vi "Simulation Time Advance.vi"(8 "error in (no error)":errorcluster, 11 "simulator":T14={"configuration"={"maxTime"=5.0, "enableVisualization"=TRUE, "Environment Definition"=path "irobotNavigationStateMachine.vi", "Record Location"=path "Simulation Record.xml", "autograde?"=TRUE, "interactive?"=FALSE, "Feedback Mode"=enum."debug navigation", "Robot State Charts"=[path "C:/Users/blueuser/Desktop/Robo Sim Berkley/cpsgrader-release-0.4/Simulators/EECS149lab/src/LabVIEW/statechart/Simulation Statechart.vi"], "statechart"=path "C:/Users/blueuser/Desktop/Robo Sim Berkley/cpsgrader-release-0.4/Simulators/EECS149lab/src/LabVIEW/statechart/Simulation Statechart.vi"}, "Statechart\ndisplay"=refnum, "first step?"=FALSE, "Robots Simulation Statecharts"=[], "Robots"=[]}) -> (0 "error out":errorcluster, 2 "Robot Sensors":T1[](array[typedef]) {"Kobuki Sensors"."Infrared" format="%02x"; "iRobot Sensors"."Infrared" format="%02x"; "accelerometer"."z axis (g)" format="%.3f"; "accelerometer"."y axis (g)" format="%.3f"; "accelerometer"."x axis (g)" format="%.3f"}, 3 "simulator":T14={"configuration"={"maxTime"=5.0, "enableVisualization"=TRUE, "Environment Definition"=path "irobotNavigationStateMachine.vi", "Record Location"=path "Simulation Record.xml", "autograde?"=TRUE, "interactive?"=FALSE, "Feedback Mode"=enum."debug navigation", "Robot State Charts"=[path "C:/Users/blueuser/Desktop/Robo Sim Berkley/cpsgrader-release-0.4/Simulators/EECS149lab/src/LabVIEW/statechart/Simulation Statechart.vi"], "statechart"=path "C:/Users/blueuser/Desktop/Robo Sim Berkley/cpsgrader-release-0.4/Simulators/EECS149lab/src/LabVIEW/statechart/Simulation Statechart.vi"}, "Statechart\ndisplay"=refnum, "first step?"=FALSE, "Robots Simulation Statecharts"=[], "Robots"=[]})   [LabVIEW 2014]
uses:
  Simulator.ctl
  CyberSim interface/Simulation Configuration.ctl
  autograder/feedbackMode.ctl
  Multi Bot Code/RobotData.ctl
  <instrlib>/DC Motor Controller/HAIOL/DC Motor Controller.lvclass
  shared/Sensors.ctl
  iRobot/Sensor/Accelerometer.ctl
  iRobot/Sensor/Sensor Group 6.ctl
  iRobot/Sensor/Bumps + Wheel Drops.ctl
  iRobot/Sensor/Buttons.ctl
  iRobot/Sensor/Charging State.ctl
  iRobot/Sensor/Charging Sources Available.ctl
  iRobot/Sensor/OI Mode.ctl
  iRobot/Sensor/Cargo Bay Digital Inputs.ctl
  iRobot/Sensor/Low-Side Driver + Wheel Overcurrent.ctl
  Kobuki/KobukiSensors.ctl
  Kobuki/Kobuki Bumps and WheelDrops.ctl
  Kobuki/Kobuki Buttons.ctl
  <vilib>/robotics/Simulator/NI_Robotics_Simulator.lvlib
panel:
  # "Electrical: charging, battery, OI mode"
  # "Sensors: bump, cliff, button, wheel drop, wall, virtual wall"
  # "Motion: distance, angle, requested velocity"
  # "Cargo Bay: I/O, overcurrent, infrared"
  # "Song"
  # "Electrical: charging, battery, OI mode"
  # "Sensors: bump, cliff, button, wheel drop, wall, virtual wall"
  # "Motion: distance, angle, requested velocity"
  # "Cargo Bay: I/O, overcurrent, infrared"
  # "Song"
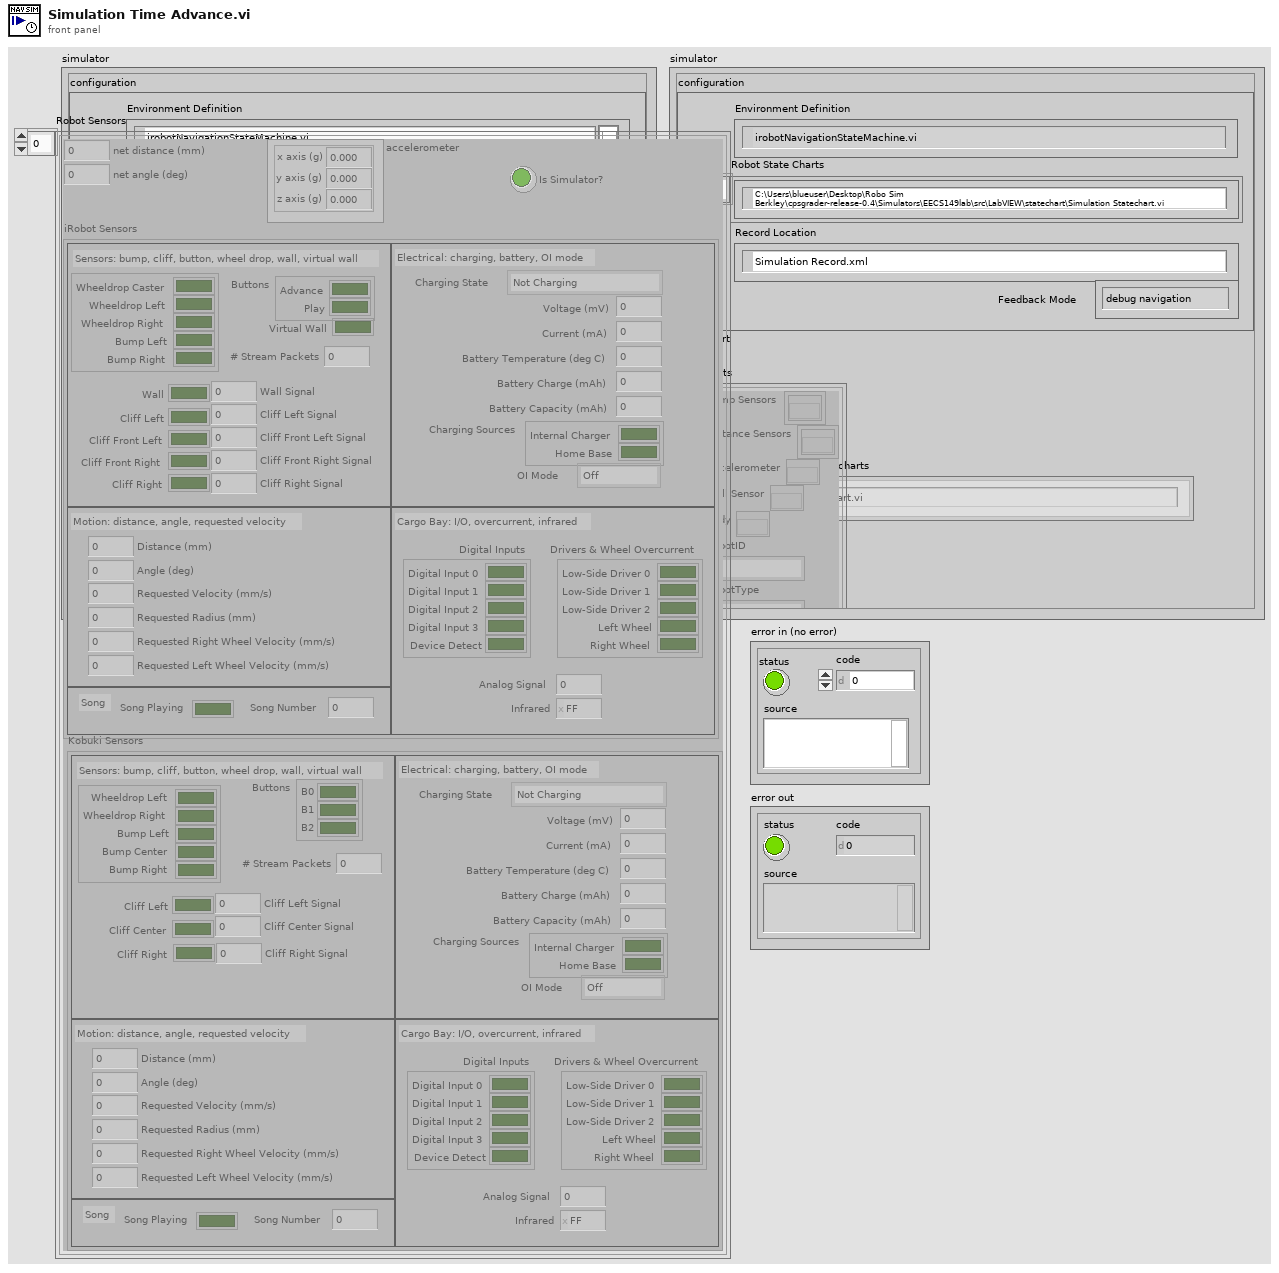
[diagram p1: front panel]
types:
  T1 = typedef "Sensors.ctl" = cluster{"net distance (mm)":i32, "net angle (deg)":i32, "accelerometer":T2, "iRobot Sensors":T3, "Is Simulator?":bool, "Kobuki Sensors":T11}
  T2 = typedef "Accelerometer.ctl" = cluster{"x axis (g)":dbl, "y axis (g)":dbl, "z axis (g)":dbl}
  T3 = typedef "Sensor Group 6.ctl" = cluster{"Bumps + Wheel Drops":T4, "Wall":bool, "Cliff Left":bool, "Cliff Front Left":bool, "Cliff Front Right":bool, "Cliff Right":bool, "Wall Signal":u16, "Cliff Left Signal":u16, "Cliff Front Left Signal":u16, "Cliff Front Right Signal":u16, "Cliff Right Signal":u16, "Buttons":T5, "Virtual Wall":bool, "# Stream Packets":u8, "Requested Velocity (mm/s)":i16, "Requested Radius (mm)":i16, "Requested Right Wheel Velocity (mm/s)":i16, "Requested Left Wheel Velocity (mm/s)":i16, "Distance (mm)":i32, "Angle (deg)":i32, "Song Playing":bool, "Song Number":u8, "Charging State":T6, "Voltage (mV)":u16, "Current (mA)":i16, "Battery Temperature (deg C)":i8, "Battery Charge (mAh)":u16, "Battery Capacity (mAh)":u16, "Charging Sources":T7, "OI Mode":T8, "Digital Inputs":T9, "Drivers & Wheel Overcurrent":T10, "Analog Signal":u16, "Infrared":u8}
  T4 = typedef "Bumps + Wheel Drops.ctl" = cluster{"Wheeldrop Caster":bool, "Wheeldrop Left":bool, "Wheeldrop Right":bool, "Bump Left":bool, "Bump Right":bool}
  T5 = typedef "Buttons.ctl" = cluster{"Advance":bool, "Play":bool}
  T6 = typedef "Charging State.ctl" = enum16{"Not Charging", "Reconditioning Charging", "Full Charging", "Trickle Charging", "Waiting", "Charging Fault Condition"}
  T7 = typedef "Charging Sources Available.ctl" = cluster{"Internal Charger":bool, "Home Base":bool}
  T8 = typedef "OI Mode.ctl" = enum16{"Off", "Passive", "Safe", "Full"}
  T9 = typedef "Cargo Bay Digital Inputs.ctl" = cluster{"Digital Input 0":bool, "Digital Input 1":bool, "Digital Input 2":bool, "Digital Input 3":bool, "Device Detect":bool}
  T10 = typedef "Low-Side Driver + Wheel Overcurrent.ctl" = cluster{"Low-Side Driver 0":bool, "Low-Side Driver 1":bool, "Low-Side Driver 2":bool, "Left Wheel":bool, "Right Wheel":bool}
  T11 = typedef "KobukiSensors.ctl" = cluster{"Bumps + Wheel Drops":T12, "Cliff Left":bool, "Cliff Center":bool, "Cliff Right":bool, "Cliff Left Signal":u16, "Cliff Center Signal":u16, "Cliff Right Signal":u16, "Buttons":T13, "# Stream Packets":u8, "Requested Velocity (mm/s)":i16, "Requested Radius (mm)":i16, "Requested Right Wheel Velocity (mm/s)":i16, "Requested Left Wheel Velocity (mm/s)":i16, "Distance (mm)":i32, "Angle (deg)":i32, "Song Playing":bool, "Song Number":u8, "Charging State":T6, "Voltage (mV)":u16, "Current (mA)":i16, "Battery Temperature (deg C)":i8, "Battery Charge (mAh)":u16, "Battery Capacity (mAh)":u16, "Charging Sources":T7, "OI Mode":T8, "Digital Inputs":T9, "Drivers & Wheel Overcurrent":T10, "Analog Signal":u16, "Infrared":u8}
  T12 = typedef "Kobuki Bumps and WheelDrops.ctl" = cluster{"Wheeldrop Left":bool, "Wheeldrop Right":bool, "Bump Left":bool, "Bump Center":bool, "Bump Right":bool}
  T13 = typedef "Kobuki Buttons.ctl" = cluster{"B0":bool, "B1":bool, "B2":bool}
  T14 = typedef "Simulator.ctl" = cluster{"configuration":T15, "Statechart\ndisplay":refnum<vi>, "first step?":bool, "Robots Simulation Statecharts":path[], "Robots":T17[]}
  T15 = typedef "Simulation Configuration.ctl" = cluster{"maxTime":sgl, "enableVisualization":bool, "Environment Definition":path, "Record Location":path, "autograde?":bool, "interactive?":bool, "Feedback Mode":T16, "Robot State Charts":path[], "statechart":path}
  T16 = typedef "feedbackMode.ctl" = enum32{"debug navigation", "debug hill climb", "autograde navigation", "autograde hill climb"}
  T17 = typedef "RobotData.ctl" = cluster{"Bump Sensors":refnum<k20>[], "Distance Sensors":refnum<k20>[], "Accelerometer":refnum<k20>, "Wall Sensor":refnum<k20>, "Body":refnum<k20>, "RobotID":string, "RobotType":string, "Left Motor":refnum<class "DC Motor Controller.lvclass">, "Right Motor":refnum<class "DC Motor Controller.lvclass">}
  T18 = typedef "Sim Sensors Feedback.ctl" = cluster{"Position":sgl[], "Position 2":dbl, "yaw":dbl, "net angle":dbl}
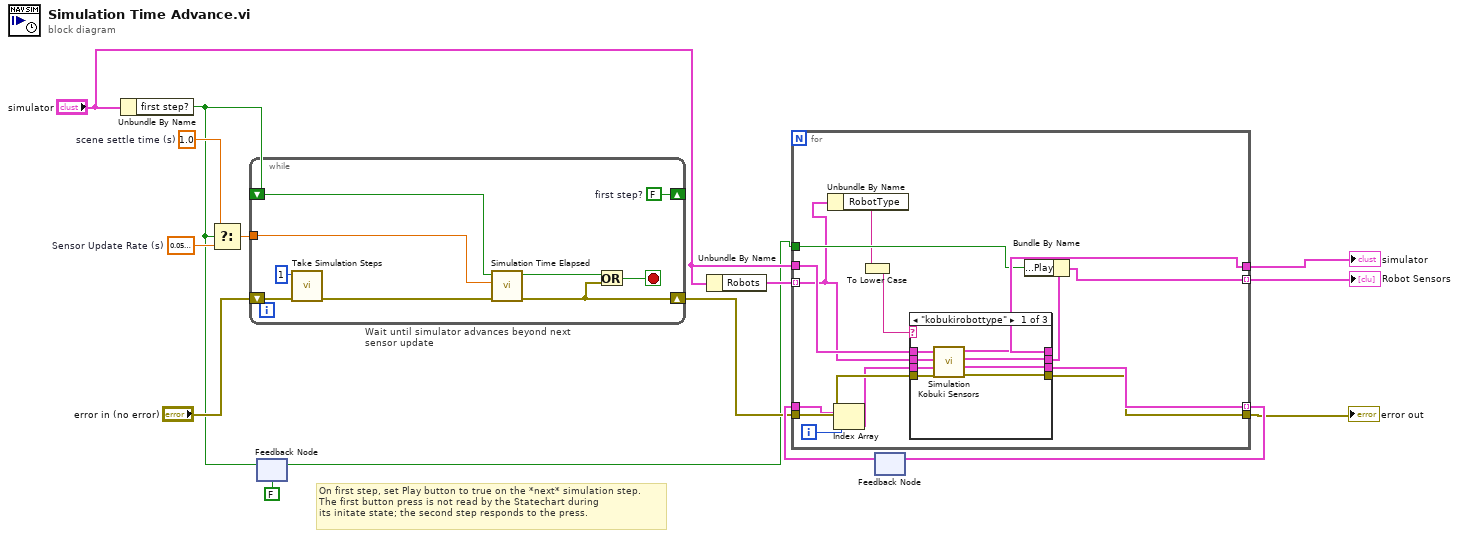
[diagram p0: block diagram]
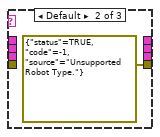
[diagram p2: hidden frame]
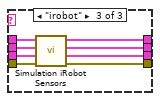
[diagram p3: hidden frame]
diagram:
  w14 = sgl 1.0  # scene settle time (s)
  w13 = sgl 0.06  # Sensor Update Rate (s)
  # "On first step, set Play button to true on the *next* simulation step.\nThe first button press is not read by the Statechart during\nits initate state; the second step responds to the press."
  n1 = Unbundle By Name("simulator") -> ("first step?"=w10:bool)
  n2 = Select(t=w14, s=w10, f=w13) -> (s? t:f=w12:sgl)
  n3 = while "Wait until simulator advances beyond next sensor update" {
    shift-right: [w20] -> w5
    shift-left: "error in (no error)" -> [w22]
    shift-right: [w17] -> _
    shift-left: w10 -> [w19]
    tunnel: w12 -> [w18]
    stop <- w21 stop-if-true
    w17 = FALSE  # first step?
    n4 = call <vilib>:"Take Simulation Steps.vi"("error in (no error)"=w22, "number of steps"=u64 1) -> ("error out"=w23:errorcluster)  [unwired: 9 in]
    n5 = call "Simulation Time Elapsed.vi"("error in (no error)"=w23, "Time Target (s)"=w18, "first step?"=w19) -> ("error out"=w20:errorcluster, "Time Elapsed?"=w16:bool)  [unwired: 6 in, 1 out]
    n6 = Or(x=w16, y=w20) -> (x .or. y?=w21:bool)
  }
  n7 = feedback #1(FALSE ("init?")) -> (w4:bool)
  n8 = feedback-in #1(w10) -> ()
  n9 = Unbundle By Name("simulator") -> ("Robots"=w9:T17[])
  n10 = feedback #2() -> (w6:T18[])  [unwired: 1 in]
  n11 = for {
    tunnel: w9 -> [w27] mode=indexing
    tunnel: "simulator" -> [w38]
    tunnel: [w37] -> w3
    tunnel: [w36] -> w7 mode=indexing
    tunnel: [w35] -> w2
    tunnel: w6 -> [w29]
    tunnel: w5 -> [w34]
    tunnel: w4 -> [w32]
    tunnel: [w31] -> w1 mode=indexing
    i -> [w30]
    n12 = Unbundle By Name(w27) -> ("RobotType"=w26:string)
    n13 = Index Array(array=w29, index=w30) -> (element=w28:T18)
    n14 = To Lower Case(string=w26) -> (all lower case string=w25:string)
    n15 = case shown="\"kobukirobottype\"" w25 {
      tunnel: w27 -> [w45 _ w55]
      tunnel: w38 -> [w46 _ w54]
      tunnel: [w41 _ w53] -> w37
      tunnel: [w39 _ w52] -> w36
      tunnel: [w42 errorcluster {"status"=TRUE, "code"=-1, "source"="Unsupported Robot Type."} ("error out") w51] -> w35
      tunnel: w34 -> [w43 _ w50]
      tunnel: [w40 _ w49] -> w33
      tunnel: w28 -> [w44 _ w48]
      frame "kobukirobottype" {
        n16 = call "Simulation Kobuki Sensors.vi"("error in"=w43, "Feedback Input"=w44, "Robot"=w45, "simulator"=w46) -> ("error out"=w42:errorcluster, "Feedback Output"=w39:T18, "sensors"=w40:T1, "simulator"=w41:T14)  [unwired: 4 in]
      }
      frame Default {
      }
      frame "irobot" {
        n17 = call "Simulation iRobot Sensors.vi"("error in"=w50, "Feedback Input"=w48, "Robot"=w55, "simulator"=w54) -> ("error out"=w51:errorcluster, "Feedback Output"=w52:T18, "sensors"=w49:T1, "simulator"=w53:T14)  [unwired: 4 in]
      }
    }
    n18 = Bundle By Name(cluster=w33, "iRobot Sensors.Buttons.Play"=w32) -> (w31:T1)
  }
  "simulator" <- w3
  "error out" <- w2
  "Robot Sensors" <- w1
  n19 = feedback-in #2(w7) -> ()
